vi "WriteToFIFOPort4.vi"(9 "String":string, 10 "loop#":i32, 11 "FPGA VI Reference Out":refnum<k20>) -> (3 "FPGA VI Reference Out 2":refnum<k20>)   [LabVIEW 2011]
uses:
  <vilib>/Utility/error.llb/Error Cluster From Error Code.vi
  <vilib>/rvi/errors/niLvFpgaAdjustHostInterfaceError.vi
  <vilib>/rvi/interface/nirviReadWriteControl/nirviReadWriteControl.xnode
  FPGA Bitfiles/SailBot_FPGATarget_ReadFromFIFOPort_B155A09E.lvbitx
  1A-FPGA/1A Code/ReadFromFIFOPort4.vi
  NiFpgaLv.dll
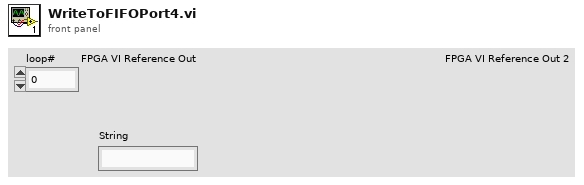
[diagram p1: front panel]
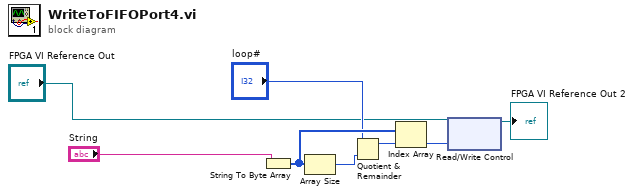
[diagram p0: block diagram]
diagram:
  n1 = String To Byte Array(string="String") -> (unsigned byte array=w5:u8[])
  n2 = Array Size(array=w5) -> (size(s)=w8:i32)
  n3 = Quotient & Remainder(x="loop#", y=w8) -> (x-y*floor(x/y)=w7:i32)  [unwired: 1 out]
  n4 = Index Array(array=w5, index=w7) -> (element=w6:u8)
  n5 = xnode "Read/Write Control"("FPGA VI Reference In"="FPGA VI Reference Out", "Data"=w6) -> ("FPGA VI Reference Out"=→"FPGA VI Reference Out 2":refnum<k20>)  [unwired: 1 in, 1 out]
